vi "ft_data_new.vi"() -> ()   [LabVIEW 2012]
uses:
  <vilib>/Utility/miscctls.llb/LVDateTimeRec.ctl
  <vilib>/addons/database/Connection.llb/DB Tools Open Connec (String).vi
  <vilib>/addons/database/NI_Database_API.lvlib
panel:
  out "s? t:f":string
  out "output cluster":T1
  in  "table 2":string
  in  "input cluster":T1
  out "text 2":string
  in  "Data":T2={"query type"="automatic", "device name"="mydevice", "Numeric"=0.0}
  in  "table":string
  out "error out":errorcluster
  out "Array 8":timestamp[](array[timestamp])
  in  "date time rec":T3
  out "Array":string[](array[string])
  in  "path":path=path "c:/"
  out "filenames":string[](array[string])
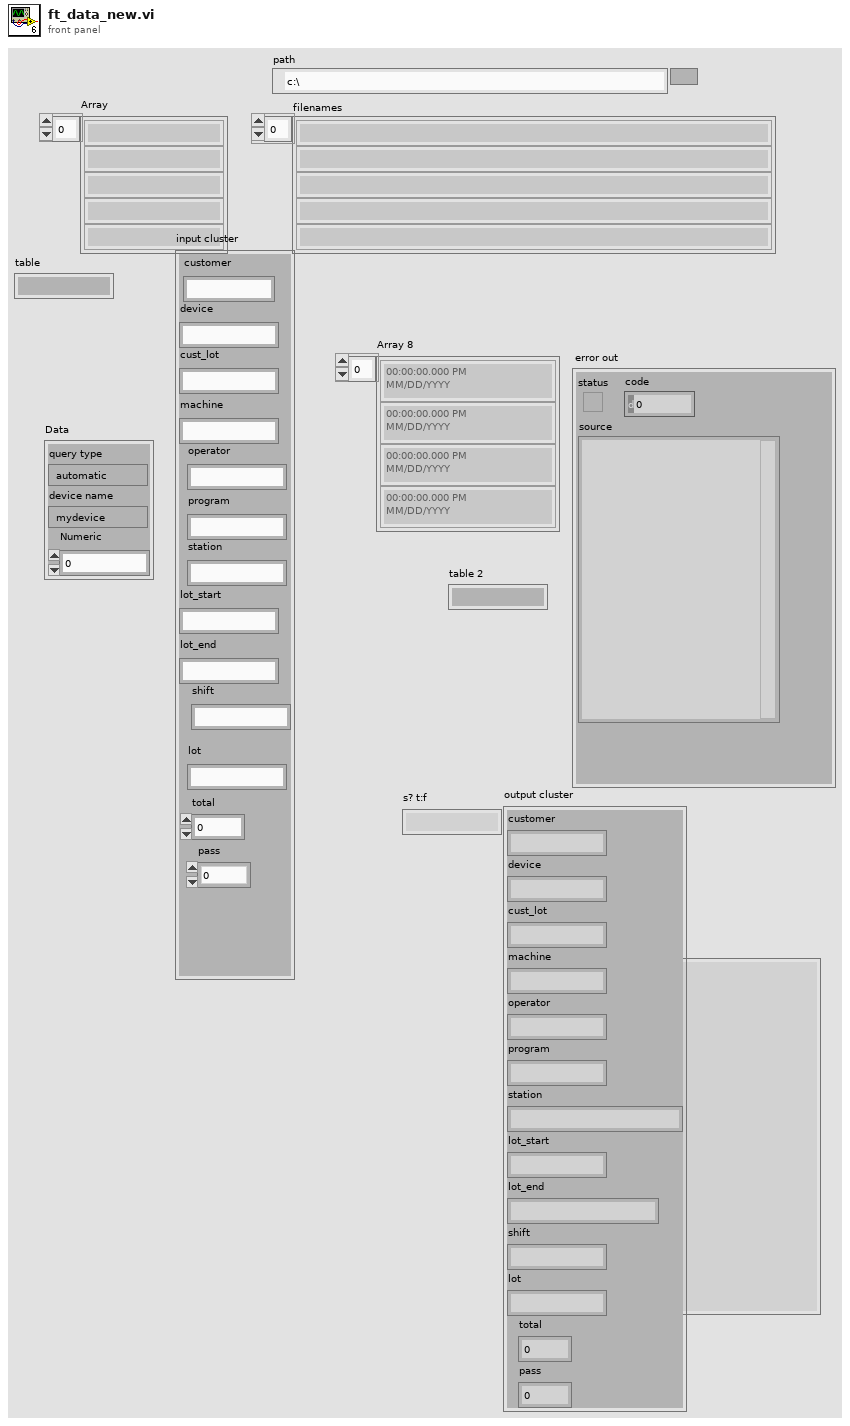
[diagram p1: front panel]
types:
  T1 = cluster{"customer":string, "device":string, "cust_lot":string, "machine":string, "operator":string, "program":string, "station":string, "lot_start":string, "lot_end":string, "shift":string, "lot":string, "total":dbl, "pass":dbl}
  T2 = cluster{"query type":string, "device name":string, "Numeric":dbl}
  T3 = typedef "LVDateTimeRec.ctl" = cluster{"fractional second":dbl, "second":i32, "minute":i32, "hour":i32, "day of month":i32, "month":i32, "year":i32, "day of week":i32, "day of year":i32, "DST":i32}
  T4 = typedef "NI_Database_API.lvlib/Conn ObjectReference.ctl" = refnum<k1>
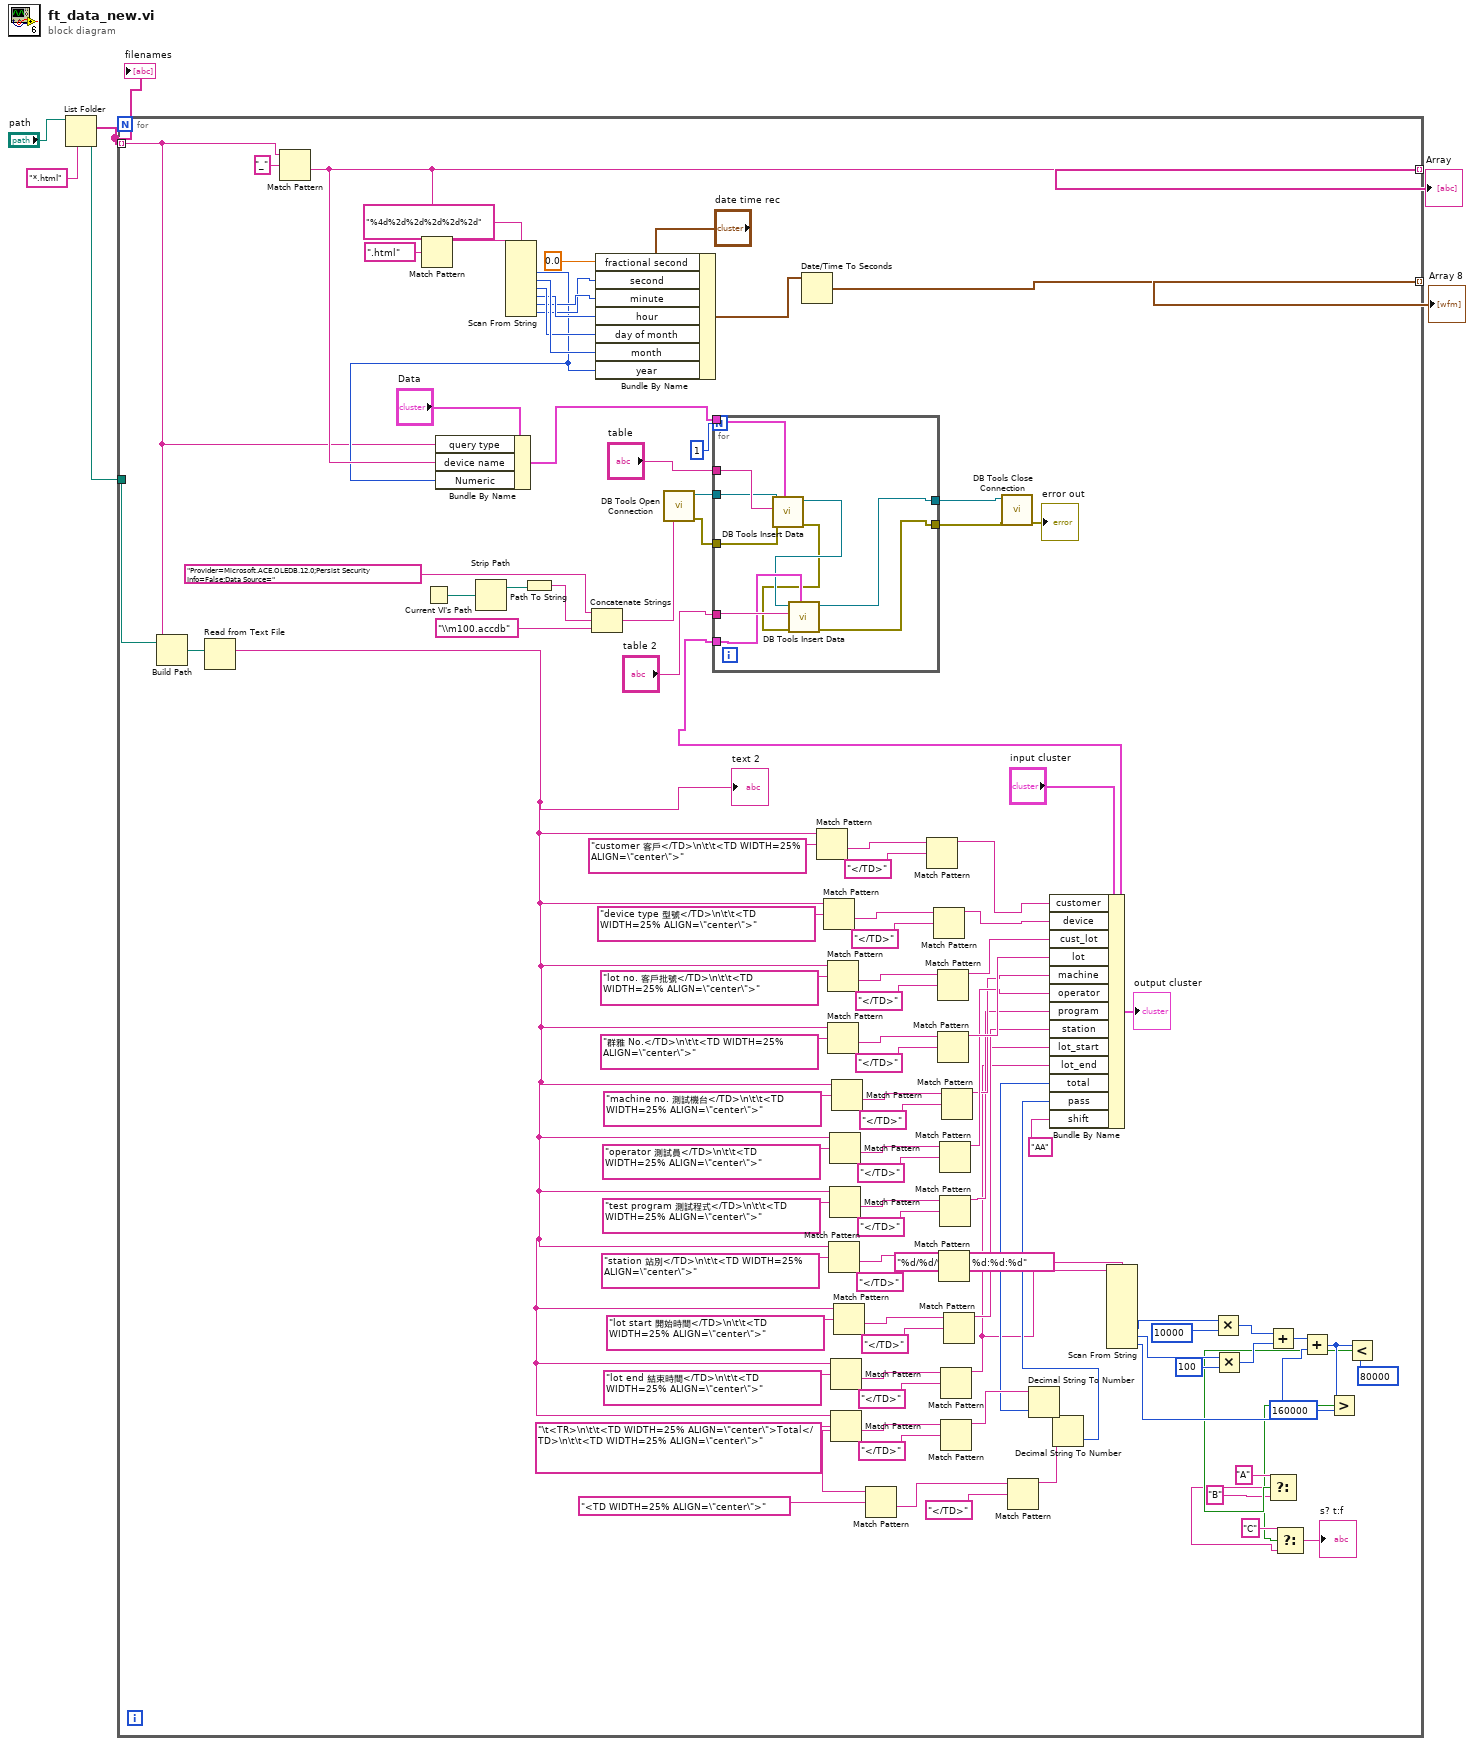
[diagram p0: block diagram]
diagram:
  n1 = List Folder(path="path", pattern="*.html") -> (path out=w1:path, filenames=w4:string[])  [unwired: 2 in, 2 out]
  "filenames" <- w4
  n2 = for {
    tunnel: w4 -> [w82] mode=indexing
    tunnel: [w85] -> w3 mode=indexing
    tunnel: [w101] -> w2 mode=indexing
    tunnel: w1 -> [w81]
    n3 = Build Path(base path=w81, name or relative path=w82) -> (appended path=w83:path)
    n4 = Read from Text File(file (use dialog)=w83) -> (text=w42:string)  [unwired: 3 in, 3 out]
    "text 2" <- w42
    n5 = Match Pattern(string=w82, regular expression="_") -> (after substring=w85:string)  [unwired: 1 in, 3 out]
    n6 = Match Pattern(string=w85, regular expression=".html") -> (before substring=w111:string)  [unwired: 1 in, 3 out]
    n7 = Current VI's Path() -> (path=w99:path)
    n8 = Strip Path(path=w99) -> (stripped path=w97:path)  [unwired: 1 out]
    n9 = Scan From String(format string="%4d%2d%2d%2d%2d%2d", input string=w111) -> (output 1=w84:i32, output 2=w107:i32, output 3=w106:i32, output 4=w105:i32, output 5=w104:i32, output 6=w103:i32)  [unwired: 8 in, 3 out]
    n10 = Bundle By Name(cluster="Data", "query type"=w82, "device name"=w85, "Numeric"=w84) -> (w86:T2)
    n11 = Path To String(path=w97) -> (string=w96:string)
    n12 = Concatenate Strings("Provider=Microsoft.ACE.OLEDB.12.0;Persist Security Info=False;Data Source=", w96, "\\m100.accdb") -> (w94:string)
    n13 = Bundle By Name(cluster="date time rec", "fractional second"=0.0, "second"=w103, "minute"=w104, "hour"=w105, "day of month"=w106, "month"=w107, "year"=w84) -> (w102:T3)
    n14 = call-poly <vilib>:"DB Tools Open Connection.vi"("connection information"=w94) -> ("error out"=w90:errorcluster, "connection reference"=w93:T4)  [unwired: 7 in]
    n15 = Date/Time To Seconds(2:w102) -> (0:w101:timestamp)  [unwired: 1 in]
    n16 = Match Pattern(string=w42, regular expression="customer 客戶</TD>\n\t\t<TD WIDTH=25% ALIGN=\"center\">") -> (after substring=w79:string)  [unwired: 1 in, 3 out]
    n17 = Match Pattern(string=w42, regular expression="device type 型號</TD>\n\t\t<TD WIDTH=25% ALIGN=\"center\">") -> (after substring=w76:string)  [unwired: 1 in, 3 out]
    n18 = Match Pattern(string=w42, regular expression="lot no. 客戶批號</TD>\n\t\t<TD WIDTH=25% ALIGN=\"center\">") -> (after substring=w73:string)  [unwired: 1 in, 3 out]
    n19 = Match Pattern(string=w42, regular expression="群雅 No.</TD>\n\t\t<TD WIDTH=25% ALIGN=\"center\">") -> (after substring=w70:string)  [unwired: 1 in, 3 out]
    n20 = Match Pattern(string=w42, regular expression="station 站別</TD>\n\t\t<TD WIDTH=25% ALIGN=\"center\">") -> (after substring=w52:string)  [unwired: 1 in, 3 out]
    n21 = Match Pattern(string=w42, regular expression="operator 測試員</TD>\n\t\t<TD WIDTH=25% ALIGN=\"center\">") -> (after substring=w58:string)  [unwired: 1 in, 3 out]
    n22 = Match Pattern(string=w42, regular expression="test program 測試程式</TD>\n\t\t<TD WIDTH=25% ALIGN=\"center\">") -> (after substring=w55:string)  [unwired: 1 in, 3 out]
    n23 = Match Pattern(string=w42, regular expression="lot end 結束時間</TD>\n\t\t<TD WIDTH=25% ALIGN=\"center\">") -> (after substring=w46:string)  [unwired: 1 in, 3 out]
    n24 = Match Pattern(string=w42, regular expression="\t<TR>\n\t\t<TD WIDTH=25% ALIGN=\"center\">Total</TD>\n\t\t<TD WIDTH=25% ALIGN=\"center\">") -> (after substring=w41:string)  [unwired: 1 in, 3 out]
    n25 = Match Pattern(string=w42, regular expression="machine no. 測試機台</TD>\n\t\t<TD WIDTH=25% ALIGN=\"center\">") -> (after substring=w61:string)  [unwired: 1 in, 3 out]
    n26 = Match Pattern(string=w42, regular expression="lot start 開始時間</TD>\n\t\t<TD WIDTH=25% ALIGN=\"center\">") -> (after substring=w49:string)  [unwired: 1 in, 3 out]
    n27 = Match Pattern(string=w41, regular expression="<TD WIDTH=25% ALIGN=\"center\">") -> (after substring=w38:string)  [unwired: 1 in, 3 out]
    n28 = Match Pattern(string=w79, regular expression="</TD>") -> (before substring=w68:string)  [unwired: 1 in, 3 out]
    n29 = Match Pattern(string=w76, regular expression="</TD>") -> (before substring=w67:string)  [unwired: 1 in, 3 out]
    n30 = Match Pattern(string=w73, regular expression="</TD>") -> (before substring=w66:string)  [unwired: 1 in, 3 out]
    n31 = Match Pattern(string=w70, regular expression="</TD>") -> (before substring=w65:string)  [unwired: 1 in, 3 out]
    n32 = Match Pattern(string=w52, regular expression="</TD>") -> (before substring=w34:string)  [unwired: 1 in, 3 out]
    n33 = Match Pattern(string=w58, regular expression="</TD>") -> (before substring=w37:string)  [unwired: 1 in, 3 out]
    n34 = Match Pattern(string=w55, regular expression="</TD>") -> (before substring=w35:string)  [unwired: 1 in, 3 out]
    n35 = Match Pattern(string=w46, regular expression="</TD>") -> (before substring=w26:string)  [unwired: 1 in, 3 out]
    n36 = Match Pattern(string=w41, regular expression="</TD>") -> (before substring=w33:string)  [unwired: 1 in, 3 out]
    n37 = Match Pattern(string=w61, regular expression="</TD>") -> (before substring=w36:string)  [unwired: 1 in, 3 out]
    n38 = Match Pattern(string=w49, regular expression="</TD>") -> (before substring=w28:string)  [unwired: 1 in, 3 out]
    n39 = Match Pattern(string=w38, regular expression="</TD>") -> (before substring=w31:string)  [unwired: 1 in, 3 out]
    n40 = Decimal String To Number(string=w33) -> (number=w32:i32)  [unwired: 2 in, 1 out]
    n41 = Decimal String To Number(string=w31) -> (number=w30:i32)  [unwired: 2 in, 1 out]
    n42 = Bundle By Name(cluster="input cluster", "customer"=w68, "device"=w67, "cust_lot"=w66, "lot"=w65, "machine"=w36, "operator"=w37, "program"=w35, "station"=w34, "lot_start"=w28, "lot_end"=w26, "total"=w32, "pass"=w30, "shift"="AA") -> (w29:T1)
    "output cluster" <- w29
    n43 = for {
      N: 1 -> [_]
      tunnel: w93 -> [w121]
      tunnel: [w116] -> w92
      tunnel: [w114] -> w91
      tunnel: w90 -> [w120]
      tunnel: "table" -> [w123]
      tunnel: w86 -> [w122]
      tunnel: "table 2" -> [w119]
      tunnel: w29 -> [w118]
      n44 = call <vilib>:"DB Tools Insert Data.vi"("data"=w122, "error in (no error)"=w120, "table"=w123, "connection reference"=w121) -> ("error out"=w115:errorcluster, "connection reference out"=w117:T4)  [unwired: 6 in]
      n45 = call <vilib>:"DB Tools Insert Data.vi"("data"=w118, "error in (no error)"=w115, "table"=w119, "connection reference"=w117) -> ("error out"=w114:errorcluster, "connection reference out"=w116:T4)  [unwired: 6 in]
    }
    n46 = call <vilib>:"DB Tools Close Connection.vi"("error in (no error)"=w91, "connection reference"=w92) -> ("error out"=→"error out":errorcluster)  [unwired: 5 in]
    n47 = Scan From String(format string="%d/%d/%d %s %d:%d:%d", input string=w26) -> (output 5=w24:i32, output 6=w22:i32, output 7=w17:i32)  [unwired: 13 in, 3 out]
    n48 = Multiply(x=w24, y=10000) -> (x*y=w20:i32)
    n49 = Multiply(x=w22, y=100) -> (x*y=w19:i32)
    n50 = Add(x=w20, y=w19) -> (x+y=w18:i32)
    n51 = Add(x=w18, y=w17) -> (x+y=w14:i32)
    n52 = Greater?(x=w14, y=160000) -> (0:w7:bool)
    n53 = Less?(x=w14, y=80000) -> (x < y?=w11:bool)
    n54 = Select(t="A", s=w11, f="B") -> (s? t:f=w9:string)
    n55 = Select(t="C", s=w7, f=w9) -> (s? t:f=→"s? t:f":string)
  }
  "Array" <- w3
  "Array 8" <- w2
